vi "rearrangetemp.vi"(9 "Points to Aquire":i32, 10 "Array in":dbl[][](array[numeric])) -> (0 "units":string[](array[string]), 1 "varnames":string[](array[string]), 3 "Array out":dbl[][](array[numeric]))   [LabVIEW 2017]
panel:
  out "String Array From File":string[][](array[string])
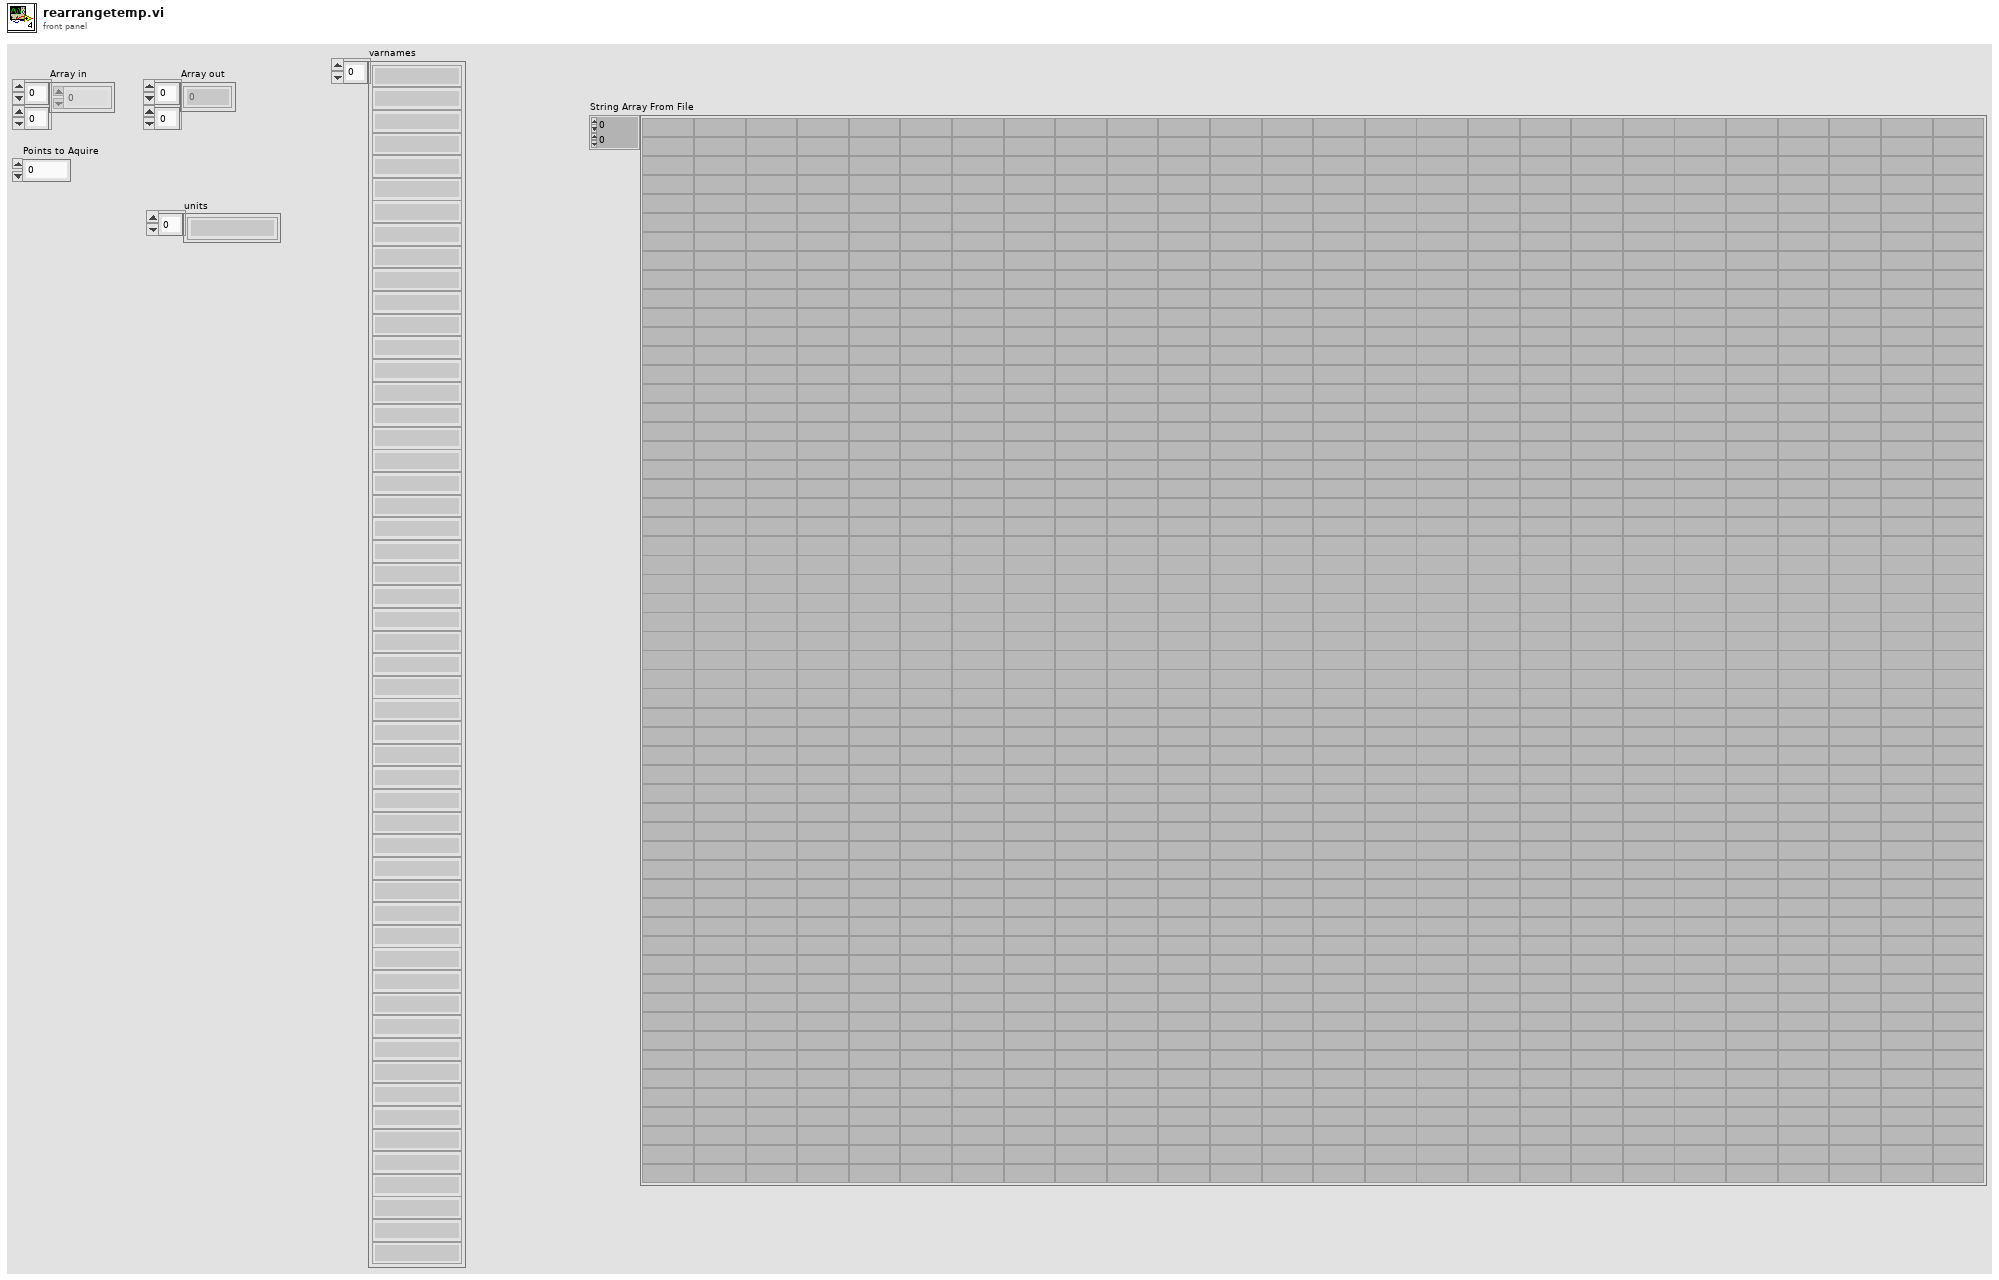
[diagram p1: front panel]
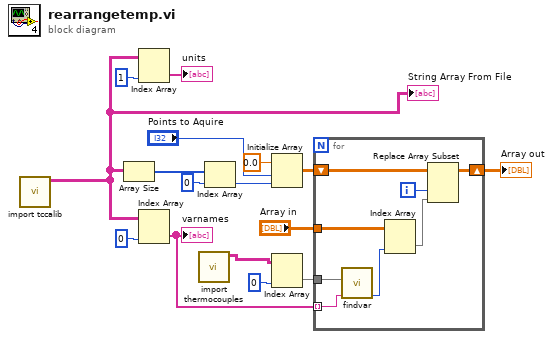
[diagram p0: block diagram]
diagram:
  n1 = call "import tccalib.vi"() -> ("String Array From File"=w2:string[][])  [unwired: 11 in]
  "String Array From File" <- w2
  n2 = Array Size(array=w2) -> (size(s)=w9:i32[])
  n3 = Index Array(array=w2, index (col)=1 ("disabled index (col)")) -> (element=→"units":string[])  [unwired: 1 in]
  n4 = Index Array(array=w2, index (col)=0 ("disabled index (col)")) -> (element=w5:string[])  [unwired: 1 in]
  "varnames" <- w5
  n5 = call "import thermocouples.vi"() -> ("String Array From File"=w1:string[][])  [unwired: 11 in]
  n6 = Index Array(array=w9, index=0) -> (element=w12:i32)
  n7 = Initialize Array(0.0 ("element"), "Points to Aquire", w12) -> (w10:dbl[][])
  n8 = Index Array(array=w1, index (col)=0 ("disabled index (col)")) -> (element=w6:string[])  [unwired: 1 in]
  n9 = for {
    tunnel: w5 -> [w24] mode=indexing
    tunnel: w6 -> [w23]
    tunnel: "Array in" -> [w19]
    shift-right: [w20] -> w14
    shift-left: w10 -> [w22]
    i -> [w21]
    n10 = call "findvar.vi"("varin"=w24, "varnames"=w23) -> ("indexno"=w18:i32)  [unwired: 8 in, 1 out]
    n11 = Index Array(array=w19, index (col)=w18) -> (element=w17:dbl[])  [unwired: 1 in]
    n12 = Replace Array Subset(array=w22, new element=w17, index (col)=w21) -> (w20:dbl[][])  [unwired: 1 in]
  }
  "Array out" <- w14
